vi "运维调试_总磷总氮.vi"() -> ()   [LabVIEW 2016, in "斯坦道总磷总氮.lvlib"]
uses:
  <vilib>/Utility/miscctls.llb/LVPointTypeDef.ctl
  <vilib>/Utility/config.llb/NI_LVConfig.lvlib
  <vilib>/ptbypt/NI_PtbyPt.lvlib
panel:
  in  "模块启用":bool
  in  "串口设置":bool
  in  "备用系数一键写入":bool
  in  "公式一键写入":bool
  in  "流程路径":path=path "C:/Users/Hsiao/Documents/斯坦道流程文件/流程.xml"
  in  "总磷总氮曲线模型":cluster{"X^2":dbl, "X":dbl, "B":dbl}(xcontrol)
  out "字符串 2":string
  in  "质控参数设置":bool
  in  "总氮自动测试量程配置":T1
  in  "总磷自动测试量程配置":T1
  out "温度2":sgl
  out "温度1":sgl
  out "ADC":sgl
  out "总氮稀释倍数":dbl
  out "固件版本号":string
  in  "数组":string[](array[string])
  in  "备用系数写入":bool
  in  "备用系数读取":bool
  in  "备用系数":T2
  in  "量程切换阈值写入":bool
  in  "量程切换阈值读取":bool
  in  "量程切换阈值":cluster{"阈值":dbl, "标液浓度":dbl}
  in  "参数下拉列表":enum16{"总磷", "总氮"}(ring)
  in  "量程下拉列表":enum16{"低量程", "高量程"}(ring)
  in  "测量模式下拉列表":enum16{"水样测量", "空白核查", "跨度核查", "标样核查", "加标回收"}(ring)
  in  "公式":cluster{"X^2":dbl, "X":dbl, "b":dbl}
  in  "写公式":bool
  in  "读公式":bool
  in  "返回":bool
  in  "设置":bool
  out "序列号":string="序列号"
  out "总氮测量数据":T3(xcontrol)
  out "总磷测量数据":T3(xcontrol)
  out "集成报警信息":string
  out "定时启动":bool
  out "总磷总氮运行状态":T4(xcontrol)
  in  "停止":bool
  in  "手动启动":bool
  in  "单步测试":bool
  in  "总磷氨氮调试":u16[](xcontrol)
  out "F3":sgl format="%#.6f"
  out "F2":sgl format="%#.6f"
  out "F1":sgl format="%#.6f"
  out "F0":sgl format="%#.6f"
  out "多列列表框":i32(listbox)
  # "参数设置"
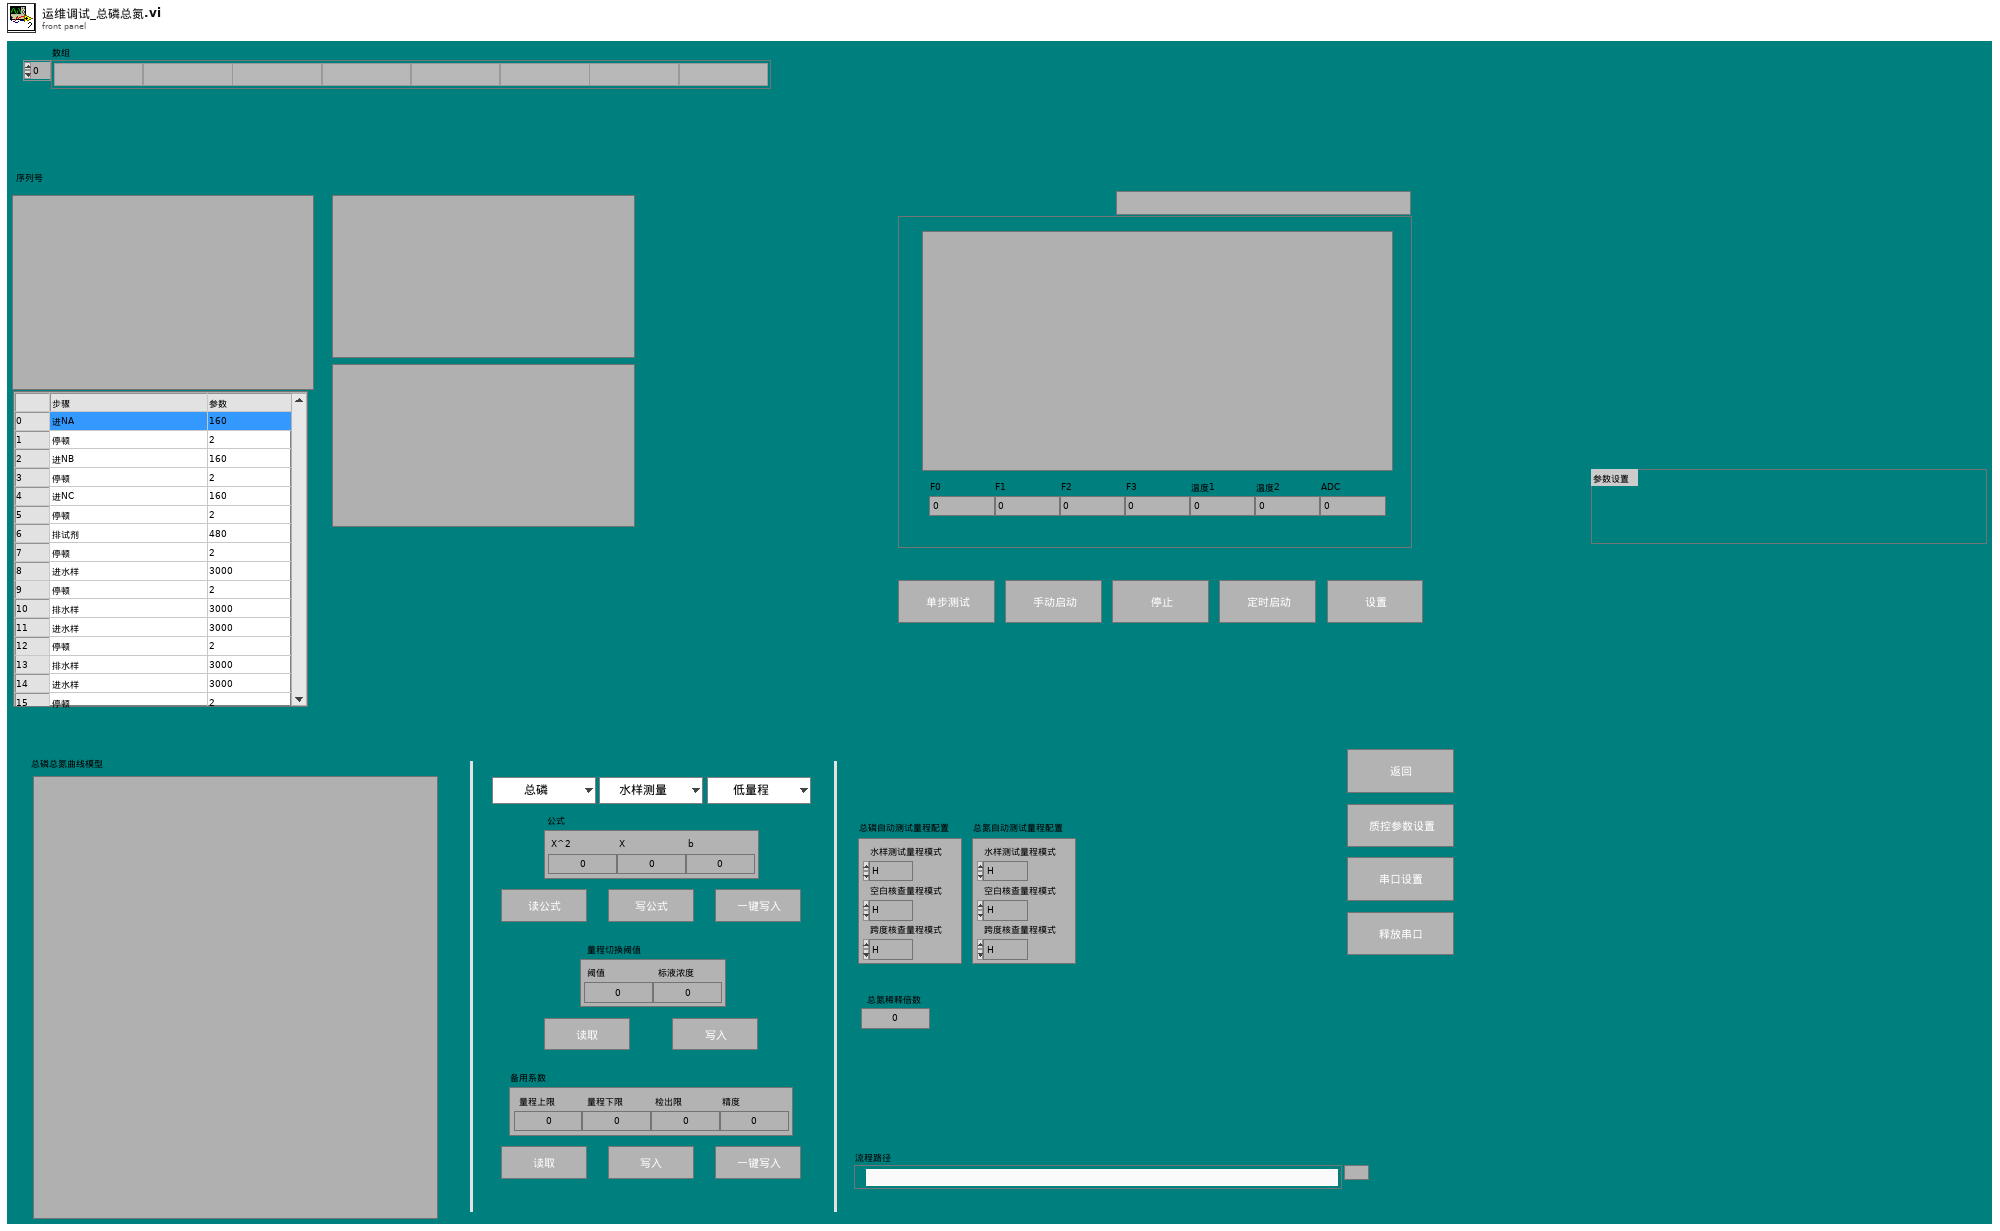
[diagram p1: front panel]
types:
  T1 = cluster{"水样测试量程模式":enum16{"H", "L", "AUTO"}, "空白核查量程模式":enum16{"H", "L", "AUTO"}, "跨度核查量程模式":enum16{"H", "L", "AUTO"}}
  T2 = cluster{"量程上限":dbl, "量程下限":dbl, "检出限":dbl, "精度":dbl}
  T3 = cluster{"flowid":u16, "测量精度":u16, "测量数据区":cluster{"因子编码":u32, "单位":u16, "标样参考值":sgl, "水样数据时间":timestamp, "水样实测值":sgl, "水样数据标识":string, "标样数据时间":timestamp, "标样实测值":sgl, "标样数据标识":string, "空白数据时间":timestamp, "空白实测值":sgl, "空白数据标识":string, "零点核查数据时间":timestamp, "零点核查实测值":sgl, "零点核查数据标识":string, "跨度核查数据时间":timestamp, "跨度核查实测值":sgl, "跨度核查数据标识":string, "加标回收数据时间":timestamp, "加标回收实测值":sgl, "加标回收数据标识":string, "平行样数据时间":timestamp, "平行样实测值":sgl, "平行样数据标识":string, "F0":sgl, "F1":sgl, "F2":sgl, "F3":sgl, "F4":sgl, "F5":sgl, "F6":sgl, "F7":sgl, "温度":sgl, "湿度":sgl, "X值":sgl}}
  T4 = cluster{"系统时间":timestamp, "工作状态":enum16{"空闲", "水样测试", "标样核查", "零点核查", "跨度核查", "空白测试", "平行样测试", "加标回收", "空白校准", "标样校准", "初始化（清洗）"}, "测量模式":enum16{"待机", "连续模式", "周期模式", "定点模式", "受控模式", "手动模式"}, "告警代码":enum16{"无告警", "缺试剂告警", "缺水样告警", "缺蒸馏水告警", "缺标液告警", "仪表漏液告警", "标定异常告警", "超量程告警", "加热异常", "低试剂预警", "超上限告警", "超下限告警", "仪表内部其他异常", "滴定异常告警", "电极异常告警", "量程切换告警", "参数设置告警", "PH电极电位异常", "电导率电极异常", "浊度光度异常", "溶解氧电极异常", "溶解氧光强异常", "温度异常告警", "PH异常告警", "溶解氧异常告警", "电导率异常告警", "浊度异常告警", "叶绿素异常告警", "藻密度异常告警", "蓝绿藻异常告警", "ORP异常告警", "氨氮异常告警", "清洁刷异常告警", "SD卡异常告警", "蓝牙异常告警", "Wifi异常告警", "流程异常告警"}, "故障代码":enum16{"无故障", "电机故障", "温度故障", "通讯故障", "滴定故障"}, "日志代码":u16, "软件版本":u16, "F0":sgl, "F1":sgl, "F2":sgl, "F3":sgl, "T":sgl, "H":sgl, "id":u16, "flowid":u16, "量程":u16, "总磷控温温度1":sgl, "营养盐控温温度2":sgl, "ADC":sgl}
  T5 = cluster{"站号":u16, "量程切换":enum32{"H", "L", "AUTO"}, "控制命令":enum16{"启动测量", "标样核查", "零点核查", "跨度核查", "空白测试", "平行样测试", "加标回收", "空白校准", "标样校准", "初始化（清洗）", "停止测试", "仪器重启", "校时", "模式设置", "测量间隔设置"}, "模式设置":enum16{"待机", "连续模式", "周期模式", "定点模式", "受控模式", "手动模式"}, "测量间隔":u16}
  T6 = enum16{"启动测量", "标样核查", "零点核查", "跨度核查", "空白测试", "平行样测试", "加标回收", "空白校准", "标样校准", "初始化（清洗）", "停止测试", "仪器重启", "校时", "模式设置", "测量间隔设置"}
  T7 = cluster{"仪器测试类型":enum16{"水样测试", "标样核查", "空白测试", "跨度核查"}, "周期设置类型":enum16{"定点启动", "间隔启动"}, "定时功能启用":bool, "定时间隔":dbl, "24H周期设置":bool[]}
  T8 = enum32{"Bad", "Idle", "Run top level", "Running"}
  T9 = typedef "LVDateTimeRec.ctl" = cluster{"秒数的小数部分":dbl, "秒":i32, "分":i32, "时":i32, "日":i32, "月":i32, "年":i32, "天数（周）":i32, "天数（年）":i32, "DST":i32}
  T10 = typedef "LVPointTypeDef.ctl" = cluster{"Horizontal":i16, "Vertical":i16}
  T11 = cluster{"因子编码":u32, "单位":u16, "标样参考值":sgl, "水样数据时间":timestamp, "水样实测值":sgl, "水样数据标识":string, "标样数据时间":timestamp, "标样实测值":sgl, "标样数据标识":string, "空白数据时间":timestamp, "空白实测值":sgl, "空白数据标识":string, "零点核查数据时间":timestamp, "零点核查实测值":sgl, "零点核查数据标识":string, "跨度核查数据时间":timestamp, "跨度核查实测值":sgl, "跨度核查数据标识":string, "加标回收数据时间":timestamp, "加标回收实测值":sgl, "加标回收数据标识":string, "平行样数据时间":timestamp, "平行样实测值":sgl, "平行样数据标识":string, "F0":sgl, "F1":sgl, "F2":sgl, "F3":sgl, "F4":sgl, "F5":sgl, "F6":sgl, "F7":sgl, "温度":sgl, "湿度":sgl, "X值":sgl}
  T12 = enum16{"空闲", "水样测试", "标样核查", "零点核查", "跨度核查", "空白测试", "平行样测试", "加标回收", "空白校准", "标样校准", "初始化（清洗）"}
  T13 = typedef "NI_LVConfig.lvlib/Config Data RefNum.ctl" = refnum<k1>
  T14 = cluster{"启动模式":enum16{"跨度核查", "水样测量", "空白核查", "标样核查", "加标回收"}, "启动参数":u16, "量程":enum16{"低量程", "高量程"}}
  T15 = cluster{"时间标识":timestamp, "设备":string, "日志信息":string, "流程参数":string}
  T16 = cluster{"时间标识":timestamp, "设备":string, "日志信息":string}
  T17 = enum16{"无告警", "缺试剂告警", "缺水样告警", "缺蒸馏水告警", "缺标液告警", "仪表漏液告警", "标定异常告警", "超量程告警", "加热异常", "低试剂预警", "超上限告警", "超下限告警", "仪表内部其他异常", "滴定异常告警", "电极异常告警", "量程切换告警", "参数设置告警", "PH电极电位异常", "电导率电极异常", "浊度光度异常", "溶解氧电极异常", "溶解氧光强异常", "温度异常告警", "PH异常告警", "溶解氧异常告警", "电导率异常告警", "浊度异常告警", "叶绿素异常告警", "藻密度异常告警", "蓝绿藻异常告警", "ORP异常告警", "氨氮异常告警", "清洁刷异常告警", "SD卡异常告警", "蓝牙异常告警", "Wifi异常告警", "流程异常告警"}
  T18 = typedef "LVRowAndColumnUnsignedTypeDef.ctl" = cluster{"Row":u32, "Column":u32}
  T19 = cluster{"总磷跨度值":dbl, "总磷零点标准液浓度":dbl, "总磷跨度标准液浓度":dbl, "总磷标准液标准浓度":dbl, "总氮跨度值":dbl, "总氮零点标准液浓度":dbl, "总氮跨度标准液浓度":dbl, "总氮标准液标准浓度":dbl}
  T20 = cluster{"确定":bool, "总磷跨度值":dbl, "总磷零点标准液浓度":dbl, "总磷跨度标准液浓度":dbl, "总磷标准液标准浓度":dbl, "总氮跨度值":dbl, "总氮零点标准液浓度":dbl, "总氮跨度标准液浓度":dbl, "总氮标准液标准浓度":dbl}
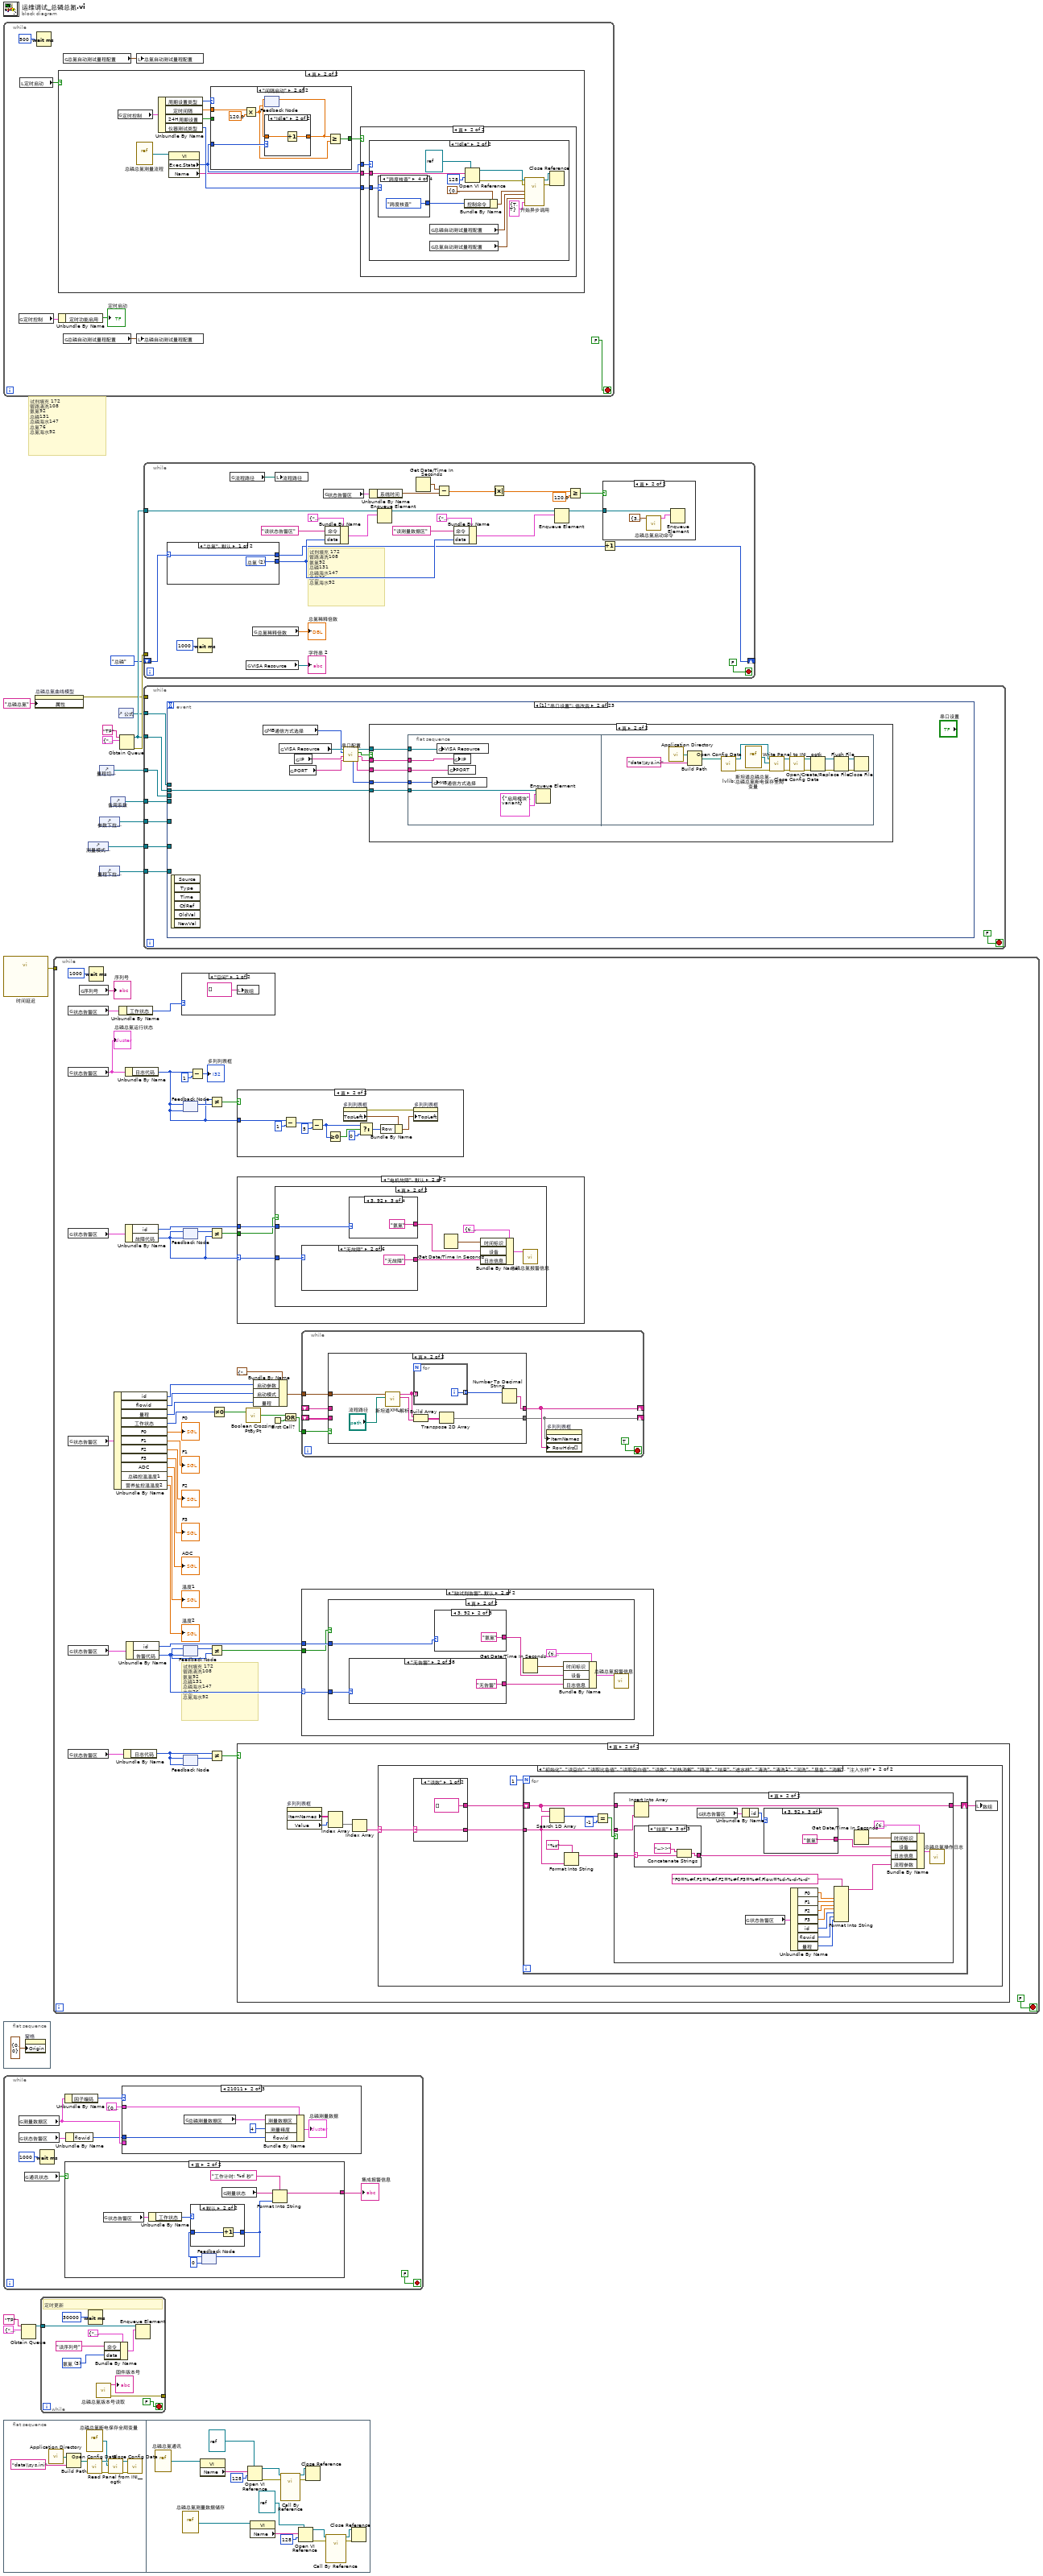
[diagram p0: block diagram]
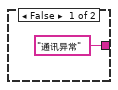
[diagram p2: hidden frame]
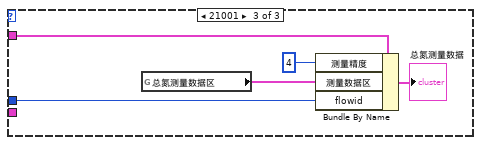
[diagram p5: hidden frame]
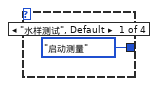
[diagram p9: hidden frame]
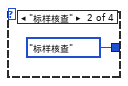
[diagram p10: hidden frame]
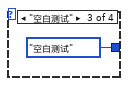
[diagram p11: hidden frame]
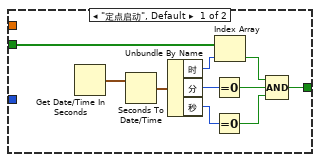
[diagram p12: hidden frame]
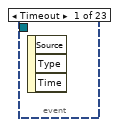
[diagram p14: hidden frame]
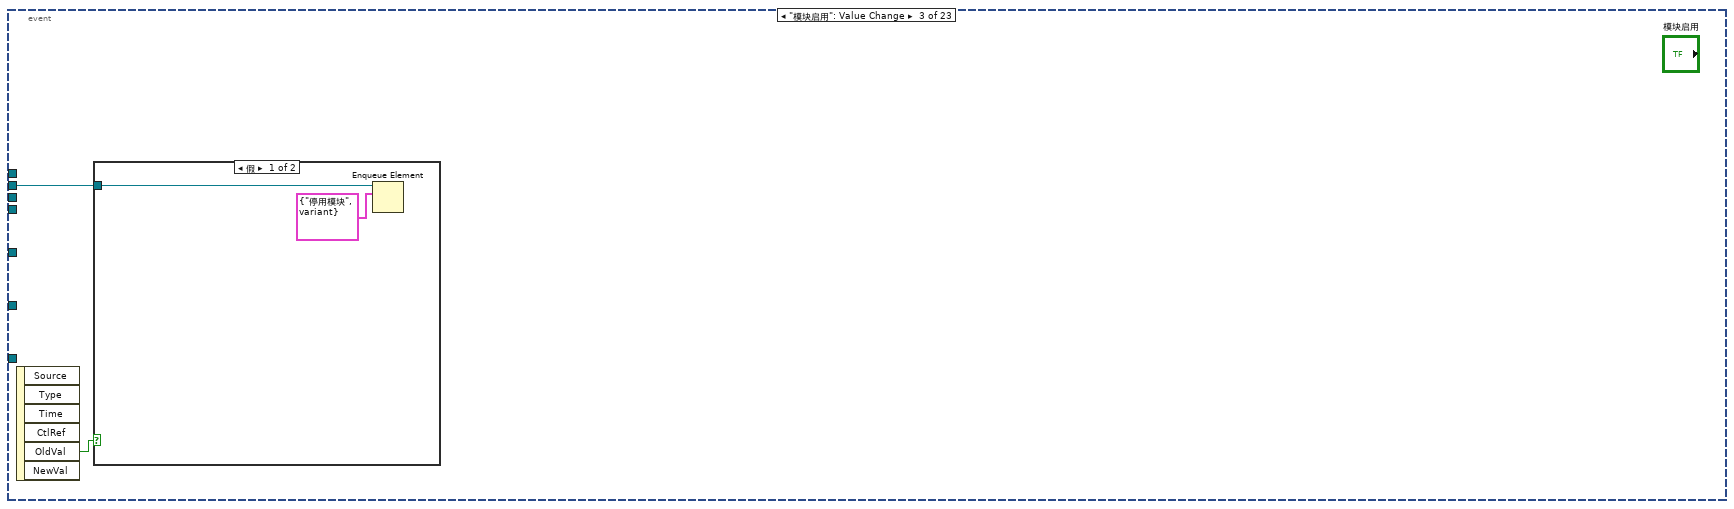
[diagram p16: hidden frame]
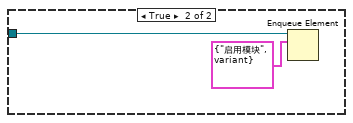
[diagram p17: hidden frame]
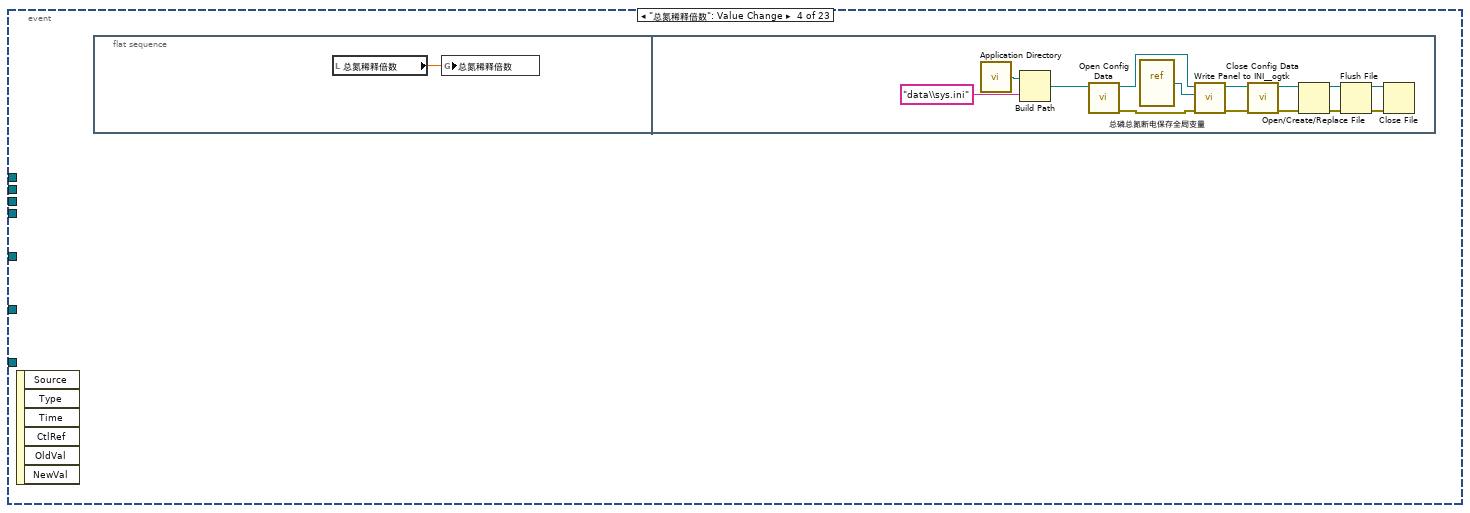
[diagram p18: hidden frame]
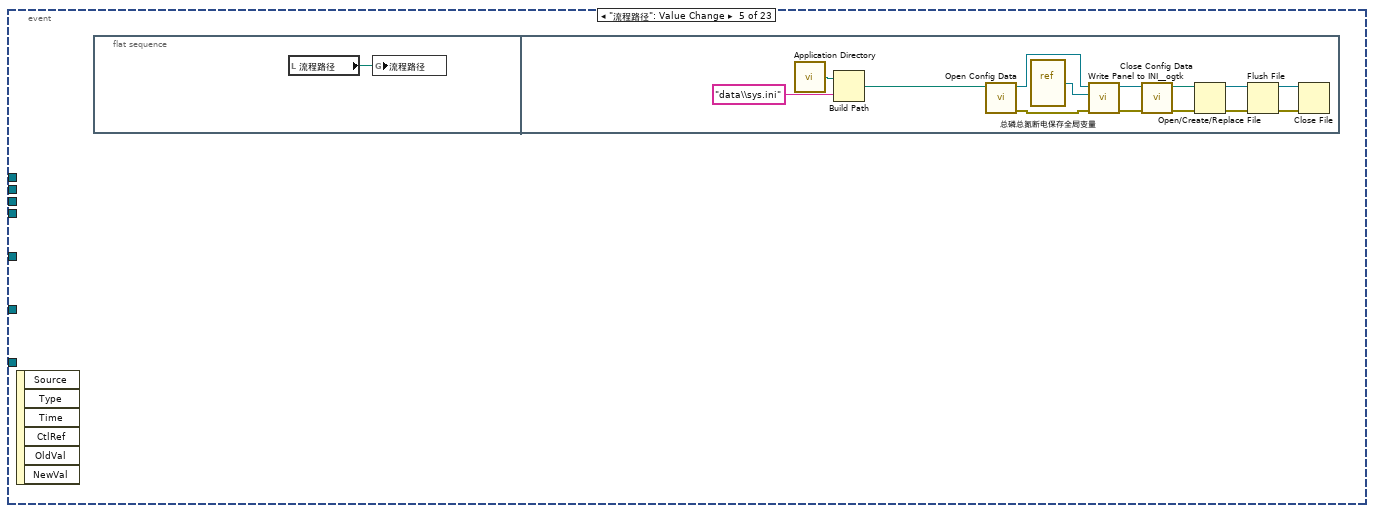
[diagram p19: hidden frame]
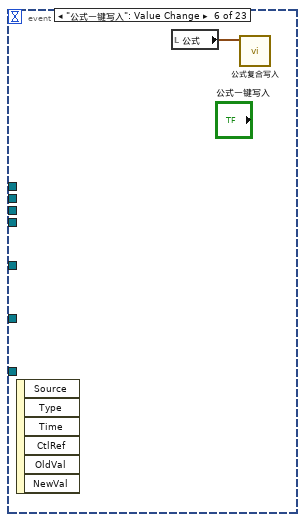
[diagram p20: hidden frame]
diagram:
  # "试剂填充 172 \n管路清洗108\n氨氮92\n总磷131\n总磷海水147\n总氮76\n总氮海水92"
  n1 = while {
    stop <- FALSE stop-if-true
    n2 = global read "总磷总氮断电保存全局变量.vi" "定时控制"() -> (w19:T7)
    n3 = local read "定时启动"() -> (w22:bool)
    n4 = Wait (ms)(milliseconds to wait=u32 500 ("等待时间（毫秒）")) -> ()  [unwired: 1 out]
    n5 = case shown="真" w22 {
      frame False {
      }
      frame True {
        n6 = global read "总磷总氮断电保存全局变量.vi" "定时控制"() -> (w33:T7)
        n7 = vi-ref "总磷总氮测量流程.vi"() -> (w28:refnum<vi>)
        n8 = Unbundle By Name(w33) -> ("周期设置类型"=w32:enum16{"定点启动", "间隔启动"}, "定时间隔"=w31:dbl, "24H周期设置"=w30:bool[], "仪器测试类型"=w27:enum16{"水样测试", "标样核查", "空白测试", "跨度核查"})
        n9 = property class="VI"(reference=w28) -> ("Exec.State"=w26:T8, "Name"=w25:string)  [unwired: 1 in, 2 out]
        n10 = case shown="\"间隔启动\"" w32 {
          tunnel: w31 -> [_ w68]
          tunnel: w30 -> [w64 _]
          tunnel: w26 -> [_ w71]
          tunnel: [w63 w66] -> w29
          frame "定点启动", Default {
            n11 = Get Date/Time In Seconds() -> (seconds since 1Jan1904=w62:timestamp)
            n12 = Seconds To Date/Time(time stamp (now)=w62) -> (date time rec=w61:T9)  [unwired: 1 in]
            n13 = Unbundle By Name(w61) -> ("时"=w60:i32, "分"=w58:i32, "秒"=w59:i32)
            n14 = Equal To 0?(x=w58) -> (x = 0?=w56:bool)
            n15 = Equal To 0?(x=w59) -> (x = 0?=w55:bool)
            n16 = Index Array(array=w64, index=w60) -> (element=w57:bool)
            n17 = Compound Arithmetic op=AND ("复合运算")(w57, w56, w55) -> (w63:bool)
          }
          frame "间隔启动" {
            n18 = Multiply(x=w68, y=120.0) -> (x*y=w65:dbl)
            n19 = feedback #1(w65) -> (w70:dbl)
            n20 = case shown="\"Idle\"" w71 {
              tunnel: w70 -> [_ w73]
              tunnel: [_ w72] -> w69
              frame "Bad", Default {
              }
              frame "Idle" {
                n21 = Increment(x=w73) -> (x+1=w72:dbl)
              }
            }
            n22 = feedback-in #1(w69) -> ()
            n23 = Greater Or Equal?(x=w69, y=w65) -> (x >= y?=w66:bool)
          }
        }
        n24 = case shown="真" w29 {
          tunnel: w25 -> [_ w36]
          tunnel: w27 -> [_ w35]
          tunnel: w26 -> [_ w34]
          frame False {
          }
          frame True {
            n25 = case shown="\"Idle\"" w34 {
              tunnel: w36 -> [_ w46]
              tunnel: w35 -> [_ w42]
              frame "Bad", Default {
              }
              frame "Idle" {
                n26 = case shown="\"跨度核查\"" w42 {
                  tunnel: [T6."启动测量" ("控制命令") T6."标样核查" ("控制命令") T6."空白测试" ("控制命令") T6."跨度核查" ("控制命令")] -> w41
                  frame "水样测试", Default {
                  }
                  frame "标样核查" {
                  }
                  frame "空白测试" {
                  }
                  frame "跨度核查" {
                  }
                }
                n27 = global read "总磷总氮断电保存全局变量.vi" "总磷自动测试量程配置"() -> (w40:T1)
                n28 = global read "总磷总氮断电保存全局变量.vi" "总氮自动测试量程配置"() -> (w39:T1)
                n29 = Bundle By Name(cluster=T5 {"站号"=0, "量程切换"=enum."H", "控制命令"=enum."启动测量", "模式设置"=enum."待机", "测量间隔"=0} ("参数"), "控制命令"=w41) -> (w43:T5)
                n30 = Open VI Reference(type specifier VI Refnum (for type only)=refnum<vi> refnum, vi path=w46, options=128 ("选项")) -> (vi reference=w47:refnum<vi>, error out=w48:errorcluster)  [unwired: 3 in]
                n31 = call-by-ref "开始异步调用"(reference=w47, error in=w48, "启动参数"=cluster{"总磷":bool, "总氮":bool} {"总磷"=TRUE, "总氮"=TRUE}, "总氮量程模式"=w39, "总磷量程模式"=w40, "参数"=w43) -> (reference out=w49:refnum<vi>, error out=w50:errorcluster)  [unwired: 8 in]
                n32 = Close Reference(reference=w49, error in (no error)=w50) -> ()  [unwired: 1 out]
              }
            }
          }
        }
      }
    }
    n33 = Unbundle By Name(w19) -> ("定时功能启用"=→"定时启动":bool)
    n34 = global read "总磷总氮断电保存全局变量.vi" "总氮自动测试量程配置"() -> (w21:T1)
    n35 = global read "总磷总氮断电保存全局变量.vi" "总磷自动测试量程配置"() -> (w20:T1)
    n36 = local write "总氮自动测试量程配置"(w21) -> ()
    n37 = local write "总磷自动测试量程配置"(w20) -> ()
  }
  n38 = call "时间延迟"() -> ("error out"=w6:errorcluster)  [unwired: 11 in]
  n39 = flat-sequence {
    frame #0 {
      n40 = property on="窗格" class="Pane"("Origin"=T10 {"Horizontal"=0, "Vertical"=0} ("原点")) -> ()  [unwired: 2 in, 2 out]
    }
  }
  n41 = while {
    stop <- FALSE stop-if-true
    n42 = global read "VAR总磷总氮全局变量.vi" "测量数据区"() -> (w81:T11)
    n43 = global read "VAR总磷总氮全局变量.vi" "状态告警区"() -> (w77:T4)
    n44 = global read "VAR总磷总氮全局变量.vi" "通讯状态"() -> (w79:bool)
    n45 = Wait (ms)(milliseconds to wait=u32 1000 ("等待时间（毫秒）")) -> ()  [unwired: 1 out]
    n46 = Unbundle By Name(w81) -> ("因子编码"=w80:u32)
    n47 = case shown="真" w79 {
      tunnel: ["通讯异常" ("集成报警信息") w86] -> w78
      frame False {
      }
      frame True {
        n48 = global read "VAR总磷总氮全局变量.vi" "状态告警区"() -> (w92:T4)
        n49 = Unbundle By Name(w92) -> ("工作状态"=w91:T12)
        n50 = feedback #2(0) -> (w89:i32)
        n51 = case shown="默认" w91 {
          tunnel: w89 -> [_ w94]
          tunnel: [_ w93] -> w87
          frame "空闲" {
          }
          frame Default {
            n52 = Increment(x=w94) -> (x+1=w93:i32)
          }
        }
        n53 = feedback-in #2(w87) -> ()
        n54 = global read "VAR总磷总氮全局变量.vi" "测量状态"() -> (w85:string)
        n55 = Format Into String(format string="工作计时: %d 秒" ("格式字符串"), initial string=w85, w87) -> (resulting string=w86:string)  [unwired: 1 in, 1 out]
      }
    }
    "集成报警信息" <- w78
    n56 = Unbundle By Name(w77) -> ("flowid"=w76:u16)
    n57 = case shown="21011" w80 {
      tunnel: w81 -> [_ _ _]
      tunnel: w76 -> [_ w97 w103]
      tunnel: T3 {"flowid"=0, "测量精度"=0, "测量数据区"={"因子编码"=0, "单位"=0, "标样参考值"=0.0, "水样数据时间"=timestamp(0 s since 1904-01-01), "水样实测值"=0.0, "水样数据标识"="", "标样数据时间"=timestamp(0 s since 1904-01-01), "标样实测值"=0.0, "标样数据标识"="", "空白数据时间"=timestamp(0 s since 1904-01-01), "空白实测值"=0.0, "空白数据标识"="", "零点核查数据时间"=timestamp(0 s since 1904-01-01), "零点核查实测值"=0.0, "零点核查数据标识"="", "跨度核查数据时间"=timestamp(0 s since 1904-01-01), "跨度核查实测值"=0.0, "跨度核查数据标识"="", "加标回收数据时间"=timestamp(0 s since 1904-01-01), "加标回收实测值"=0.0, "加标回收数据标识"="", "平行样数据时间"=timestamp(0 s since 1904-01-01), "平行样实测值"=0.0, "平行样数据标识"="", "F0"=0.0, "F1"=0.0, "F2"=0.0, "F3"=0.0, "F4"=0.0, "F5"=0.0, "F6"=0.0, "F7"=0.0, "温度"=0.0, "湿度"=0.0, "X值"=0.0}} ("总氮测量数据") -> [_ w96 w102]
      frame Default {
      }
      frame 21011 {
        n58 = global read "VAR总磷总氮全局变量.vi" "总磷测量数据区"() -> (w95:T11)
        n59 = Bundle By Name(cluster=w96, "测量数据区"=w95, "测量精度"=u16 4, "flowid"=w97) -> (→"总磷测量数据":T3)
      }
      frame 21001 {
        n60 = global read "VAR总磷总氮全局变量.vi" "总氮测量数据区"() -> (w100:T11)
        n61 = Bundle By Name(cluster=w102, "测量精度"=u16 4, "测量数据区"=w100, "flowid"=w103) -> (→"总氮测量数据":T3)
      }
    }
  }
  n62 = flat-sequence {
    frame #0 {
      n63 = call <vilib>:"Application Directory.vi"() -> ("Application Directory"=w112:path)
      n64 = Build Path(base path=w112, name or relative path="data\\sys.ini" ("名称或相对路径")) -> (appended path=w110:path)
      n65 = vi-ref "总磷总氮断电保存全局变量.vi"() -> (w108:refnum<vi>)
      n66 = call <vilib>:"Open Config Data.vi"("configuration file path"=w110) -> ("error out"=w106:errorcluster, "refnum"=w109:T13)  [unwired: 8 in, 1 out]
      n67 = call <userlib>:"Read Panel from INI__ogtk.vi"("error in (no error)"=w106, "VI ref"=w108, "refnum"=w109) -> ("error out"=w105:errorcluster, "refnum out"=w107:T13)  [unwired: 7 in]
      n68 = call <vilib>:"Close Config Data.vi"("error in (no error)"=w105, "refnum"=w107) -> ()  [unwired: 8 in, 2 out]
    }
    frame #1 {
      n69 = vi-ref "总磷总氮通讯.vi"() -> (w128:refnum<vi>)
      n70 = vi-ref "总磷总氮测量数据储存.vi"() -> (w120:refnum<vi>)
      n71 = property class="VI"(reference=w128) -> ("Name"=w127:string)  [unwired: 1 in, 2 out]
      n72 = Open VI Reference(type specifier VI Refnum (for type only)=refnum<vi> refnum, vi path=w127, options=128 ("选项")) -> (vi reference=w125:refnum<vi>, error out=w123:errorcluster)  [unwired: 3 in]
      n73 = property class="VI"(reference=w120) -> ("Name"=w113:string)  [unwired: 1 in, 2 out]
      n74 = call-by-ref "?"(reference=w125, error in=w123) -> (reference out=w121:refnum<vi>, error out=w122:errorcluster)  [unwired: 12 in]
      n75 = Open VI Reference(type specifier VI Refnum (for type only)=refnum<vi> refnum, vi path=w113, options=128 ("选项")) -> (vi reference=w115:refnum<vi>, error out=w117:errorcluster)  [unwired: 3 in]
      n76 = Close Reference(reference=w121, error in (no error)=w122) -> ()  [unwired: 1 out]
      n77 = call-by-ref "?"(reference=w115, error in=w117) -> (reference out=w119:refnum<vi>, error out=w118:errorcluster)  [unwired: 12 in]
      n78 = Close Reference(reference=w119, error in (no error)=w118) -> ()  [unwired: 1 out]
    }
  }
  n79 = Obtain Queue(name (unnamed)="TP" ("名称（未命名）"), element data type=cluster{"命令":string, "data":variant} {"命令"="", "data"=variant}) -> (queue out=w3:refnum<queue>)  [unwired: 3 in, 2 out]
  n80 = property on="总磷总氮曲线模型" class="曲线模型 (严格)"("属性"="总磷总氮" ("调用模块名称属性")) -> (error out=w1:errorcluster)  [unwired: 2 in, 1 out]
  n81 = while {
    tunnel: w3 -> [w133]
    tunnel: [w129] -> _
    stop <- FALSE stop-if-true
    w134 = u16 3 items=["总磷"=1, "氨氮"=3] ("站号")
    # "定时更新"
    n82 = Wait (ms)(milliseconds to wait=u32 30000 ("等待时间（毫秒）")) -> ()  [unwired: 1 out]
    n83 = call "总磷总氮版本号读取.vi"() -> ("error out"=w129:errorcluster, "固件版本号"=→"固件版本号":string)  [unwired: 10 in]
    n84 = Bundle By Name(cluster=cluster{"命令":string, "data":variant} {"命令"="", "data"=variant} ("元素"), "命令"="读序列号", "data"=w134) -> (w132:cluster{"命令":string, "data":variant})
    n85 = Enqueue Element(queue=w133, element=w132) -> ()  [unwired: 2 in, 3 out]
  }
  n86 = while {
    tunnel: w6 -> [_]
    stop <- FALSE stop-if-true
    # "试剂填充 172 \n管路清洗108\n氨氮92\n总磷131\n总磷海水147\n总氮76\n总氮海水92"
    n87 = global read "VAR总磷总氮全局变量.vi" "状态告警区"() -> (w152:T4)
    n88 = global read "VAR总磷总氮全局变量.vi" "状态告警区"() -> (w165:T4)
    "总磷总氮运行状态" <- w165
    n89 = global read "VAR总磷总氮全局变量.vi" "状态告警区"() -> (w157:T4)
    n90 = global read "VAR总磷总氮全局变量.vi" "状态告警区"() -> (w173:T4)
    n91 = global read "VAR总磷总氮全局变量.vi" "状态告警区"() -> (w162:T4)
    n92 = global read "VAR总磷总氮全局变量.vi" "状态告警区"() -> (w149:T4)
    n93 = global read "VAR总磷总氮全局变量.vi" "序列号"() -> (→"序列号":string)
    n94 = Wait (ms)(milliseconds to wait=u32 1000 ("等待时间（毫秒）")) -> ()  [unwired: 1 out]
    n95 = Unbundle By Name(w173) -> ("id"=w170:u16, "flowid"=w172:u16, "量程"=w171:u16, "工作状态"=w139:T12, "F0"=→"F0":sgl, "F1"=→"F1":sgl, "F2"=→"F2":sgl, "F3"=→"F3":sgl, "ADC"=→"ADC":sgl, "总磷控温温度1"=→"温度1":sgl, "营养盐控温温度2"=→"温度2":sgl)
    n96 = Unbundle By Name(w152) -> ("工作状态"=w151:T12)
    n97 = Unbundle By Name(w149) -> ("日志代码"=w148:u16)
    n98 = Unbundle By Name(w165) -> ("日志代码"=w145:u16)
    n99 = Unbundle By Name(w157) -> ("id"=w156:u16, "故障代码"=w153:enum16{"无故障", "电机故障", "温度故障", "通讯故障", "滴定故障"})
    n100 = Unbundle By Name(w162) -> ("id"=w161:u16, "告警代码"=w158:T17)
    n101 = case shown="\"空闲\"" w151 {
      frame "空闲" {
        n102 = local write "数组"(string[] [] ("数组")) -> ()
      }
      frame "水样测试", Default {
      }
    }
    n103 = feedback-in #3(w145) -> ()
    n104 = feedback #3(w145) -> (w178:u16)
    n105 = feedback #4(w153) -> (w154:enum16{"无故障", "电机故障", "温度故障", "通讯故障", "滴定故障"})
    n106 = feedback-in #4(w153) -> ()
    n107 = feedback #5(w158) -> (w159:T17)
    n108 = feedback-in #5(w158) -> ()
    n109 = feedback #6(w148) -> (w150:u16)
    n110 = feedback-in #6(w148) -> ()
    n111 = Subtract(x=w145, y=1) -> (x-y=→"多列列表框":i32)
    n112 = Not Equal?(x=w145, y=w178) -> (x != y?=w177:bool)
    n113 = Not Equal?(x=w154, y=w153) -> (x != y?=w155:bool)
    n114 = Not Equal?(x=w159, y=w158) -> (x != y?=w160:bool)
    n115 = Not Equal?(x=w148, y=w150) -> (x != y?=w147:bool)
    n116 = Not Equal To 0?(x=w139) -> (x != 0?=w175:bool)
    n117 = case shown="真" w177 {
      tunnel: w145 -> [_ w331]
      frame False {
      }
      frame True {
        n118 = Subtract(x=w331, y=1) -> (x-y=w329:i32)
        n119 = Subtract(x=w329, y=5) -> (x-y=w333:i32)
        n120 = Greater Or Equal To 0?(x=w333) -> (x >= 0?=w332:bool)
        n121 = property on="多列列表框" class="MCListbox (严格)"() -> (error out=w337:errorcluster, "TopLeft"=w338:T18)  [unwired: 2 in, 1 out]
        n122 = Select(t=w333, s=w332, f=0) -> (s? t:f=w334:i32)
        n123 = Bundle By Name(cluster=w338, "Row"=w334) -> (w339:T18)
        n124 = property on="多列列表框" class="MCListbox (严格)"(error in=w337, "TopLeft"=w339) -> ()  [unwired: 1 in, 2 out]
      }
    }
    n125 = case shown="\"电机故障\", 默认" w153 {
      selector: w153 -> [_ w236]
      tunnel: w156 -> [_ w237]
      tunnel: w155 -> [_ w235]
      frame "无故障" {
      }
      frame "电机故障", Default {
        n126 = case shown="真" w235 {
          tunnel: w237 -> [_ w244]
          tunnel: w236 -> [_ w239]
          frame False {
          }
          frame True {
            n127 = case shown="\"无故障\"" w239 {
              selector: w239 -> [w246 _ _ _ _ _]
              tunnel: [w245 "无故障" "电机故障" "温度故障" "通讯故障" "滴定故障"] -> w238
              frame Default {
                n128 = Format Into String(format string="%d" ("格式字符串"), initial string="未知" ("工作状态"), w246) -> (resulting string=w245:string)  [unwired: 1 in, 1 out]
              }
              frame "无故障" {
              }
              frame "电机故障" {
              }
              frame "温度故障" {
              }
              frame "通讯故障" {
              }
              frame "滴定故障" {
              }
            }
            n129 = case shown="3, 92" w244 {
              tunnel: [_ "总磷" ("table输入") "氨氮" ("table输入") "总氮" ("table输入")] -> w240
              frame Default {
              }
              frame 1, 131 {
              }
              frame 3, 92 {
              }
              frame 2, 76 {
              }
            }
            n130 = Get Date/Time In Seconds() -> (seconds since 1Jan1904=w241:timestamp)
            n131 = Bundle By Name(cluster=T16 {"时间标识"=timestamp(0 s since 1904-01-01), "设备"="", "日志信息"=""} ("data in"), "时间标识"=w241, "设备"=w240, "日志信息"=w238) -> (w242:T16)
            n132 = call "总磷总氮报警信息.vi"("data in"=w242) -> ()  [unwired: 11 in]
          }
        }
      }
    }
    n133 = case shown="真" w147 {
      frame False {
      }
      frame True {
        n134 = property on="多列列表框" class="MCListbox (严格)"() -> ("ItemNames"=w184:string[][], "Value"=w185:i32)  [unwired: 2 in, 2 out]
        n135 = Index Array(array=w184, index (row)=w185) -> (element=w183:string[])  [unwired: 1 in]
        n136 = Index Array(array=w183) -> (element=w182:string)  [unwired: 1 in]
        n137 = case shown="\"初始化\", \"读空白\", \"读取比色值\", \"读取空白值\", \"读数\", \"加热消解\", \"降温\", \"结束\", \"进水样\", \"清洗\", \"清洗1\", \"润洗\", \"显色\", \"消解\", \"注入水样\"" w182 {
          selector: w182 -> [_ w188]
          frame Default {
          }
          frame "初始化", "读空白", "读取比色值", "读取空白值", "读数", "加热消解", "降温", "结束", "进水样", "清洗", "清洗1", "润洗", "显色", "消解", "注入水样" {
            n138 = case shown="\"读数\"" w188 {
              selector: w188 -> [w192 w194]
              tunnel: [w192 w194] -> w187
              tunnel: [string[] [] ("数组") "数组"] -> w186
              frame "读数" {
              }
              frame Default {
              }
            }
            n139 = for {
              N: 1 -> [_]
              tunnel: w187 -> [w196]
              shift-right: [w195] -> w189
              shift-left: w186 -> [w197]
              n140 = Search 1D Array(1D array=w197, element=w196) -> (index of element=w200:i32)  [unwired: 1 in]
              n141 = Format Into String(format string="%s" ("格式字符串"), w196) -> (resulting string=w201:string)  [unwired: 2 in, 1 out]
              n142 = Equal?(x=w200, y=-1) -> (x = y?=w198:bool)
              n143 = case shown="真" w198 {
                tunnel: w201 -> [_ w205]
                tunnel: w197 -> [w203 w209]
                tunnel: w196 -> [_ w208]
                tunnel: [w203 w207] -> w195
                frame False {
                }
                frame True {
                  n144 = Insert Into Array(array=w209, new element=w208) -> (w207:string[])  [unwired: 1 in]
                  n145 = case shown="\"结束\"" w205 {
                    selector: w205 -> [w225 w228 w231]
                    tunnel: [w225 w227 w230] -> w204
                    frame Default {
                    }
                    frame "初始化" {
                      n146 = Concatenate Strings("-->>" ("字符串"), w228) -> (w227:string)
                    }
                    frame "结束" {
                      n147 = Concatenate Strings("-->>" ("字符串"), w231) -> (w230:string)
                    }
                  }
                  n148 = global read "VAR总磷总氮全局变量.vi" "状态告警区"() -> (w224:T4)
                  n149 = Unbundle By Name(w224) -> ("id"=w223:u16)
                  n150 = global read "VAR总磷总氮全局变量.vi" "状态告警区"() -> (w219:T4)
                  n151 = case shown="3, 92" w223 {
                    tunnel: [_ "总磷" ("table输入") "氨氮" ("table输入") "总氮" ("table输入")] -> w221
                    frame Default {
                    }
                    frame 1, 131 {
                    }
                    frame 3, 92 {
                    }
                    frame 2, 76 {
                    }
                  }
                  n152 = Unbundle By Name(w219) -> ("F0"=w216:sgl, "F1"=w215:sgl, "F2"=w214:sgl, "F3"=w213:sgl, "id"=w212:u16, "flowid"=w211:u16, "量程"=w210:u16)
                  n153 = Format Into String(format string="F0=%#f,F1=%#f,F2=%#f,F3=%#f,Flow=%d-%-d-%-d" ("格式字符串"), w216, w215, w214, w213, w212, w211, w210) -> (resulting string=w217:string)  [unwired: 2 in, 1 out]
                  n154 = Get Date/Time In Seconds() -> (seconds since 1Jan1904=w220:timestamp)
                  n155 = Bundle By Name(cluster=T15 {"时间标识"=timestamp(0 s since 1904-01-01), "设备"="", "日志信息"="", "流程参数"=""} ("data in"), "时间标识"=w220, "设备"=w221, "日志信息"=w204, "流程参数"=w217) -> (w222:T15)
                  n156 = call "总磷总氮操作日志.vi"("data in"=w222) -> ()  [unwired: 11 in]
                }
              }
            }
            n157 = local write "数组"(w189) -> ()
          }
        }
      }
    }
    n158 = call <vilib>:"Boolean Crossing PtByPt.vi"("input"=w175) -> ("crossing"=w138:bool)  [unwired: 2 in]
    n159 = Bundle By Name(cluster=T14 {"启动模式"=enum."跨度核查", "启动参数"=1, "量程"=enum."低量程"} ("参数簇"), "启动参数"=w170, "启动模式"=w172, "量程"=w171) -> (w164:T14)
    n160 = First Call?() -> (First Call?: T/F=w176:bool)
    n161 = Or(x=w138, y=w176) -> (x .or. y?=w174:bool)
    n162 = while {
      tunnel: w174 -> [w317]
      tunnel: w164 -> [w316]
      shift-right: [w311] -> _
      shift-left: _ -> [w313]
      shift-right: [w312] -> _
      shift-left: _ -> [w314]
      stop <- TRUE stop-if-true
      n163 = case shown="真" w317 {
        tunnel: [w319 w327] -> w312
        tunnel: [w318 w326] -> w311
        tunnel: w316 -> [_ w321]
        tunnel: w314 -> [w319 _]
        tunnel: w313 -> [w318 _]
        frame False {
        }
        frame True {
          n164 = call "斯坦道XML解析.vi"("添加的路径"="流程路径", "参数簇"=w321) -> ("步骤时间"=w322:string[], "步骤名"=w324:string[])  [unwired: 8 in]
          n165 = for {
            tunnel: w324 -> [_] mode=indexing
            tunnel: [w328] -> w325 mode=indexing
            i -> [w328]
          }
          n166 = Build Array(w324, w322) -> (w323:string[][])
          n167 = Transpose 2D Array(2D array=w323) -> (transposed array=w326:string[][])
          n168 = Number To Decimal String(number=w325) -> (decimal integer string=w327:string[])  [unwired: 1 in]
        }
      }
      n169 = property on="多列列表框" class="MCListbox (严格)"("ItemNames"=w311, "RowHdrs[]"=w312) -> ()  [unwired: 2 in, 2 out]
    }
    n170 = case shown="\"缺试剂告警\", 默认" w158 {
      selector: w158 -> [_ w258]
      tunnel: w161 -> [_ w259]
      tunnel: w160 -> [_ w257]
      frame "无告警" {
      }
      frame "缺试剂告警", Default {
        n171 = case shown="真" w257 {
          tunnel: w259 -> [_ w266]
          tunnel: w258 -> [_ w260]
          frame False {
          }
          frame True {
            n172 = case shown="\"无告警\"" w260 {
              selector: w260 -> [w268 _ _ _ _ _ _ _ _ _ _ _ _ _ _ _ _ _ _ _ _ _ _ _ _ _ _ _ _ _ _ _ _ _ _ _ _ _]
              tunnel: [w267 "无告警" "缺试剂告警" "缺水样告警" "缺蒸馏水告警" "缺标液告警" "仪表漏液告警" "标定异常告警" "超量程告警" "加热异常" "低试剂预警" "超上限告警" "超下限告警" "仪表内部其他异常" "滴定异常告警" "电极异常告警" "量程切换告警" "参数设置告警" "PH电极电位异常" "电导率电极异常" "浊度光度异常" "溶解氧电极异常" "溶解氧光强异常" "温度异常告警" "PH异常告警" "溶解氧异常告警" "电导率异常告警" "浊度异常告警" "叶绿素异常告警" "藻密度异常告警" "蓝绿藻异常告警" "ORP异常告警" "氨氮异常告警" "清洁刷异常告警" "SD卡异常告警" "蓝牙异常告警" "WiFi异常告警" "流程异常告警"] -> w261
              frame Default {
                n173 = Format Into String(format string="%d" ("格式字符串"), initial string="未知" ("工作状态"), w268) -> (resulting string=w267:string)  [unwired: 1 in, 1 out]
              }
              frame "无告警" {
              }
              frame "缺试剂告警" {
              }
              frame "缺水样告警" {
              }
              frame "缺蒸馏水告警" {
              }
              frame "缺标液告警" {
              }
              frame "仪表漏液告警" {
              }
              frame "标定异常告警" {
              }
              frame "超量程告警" {
              }
              frame "加热异常" {
              }
              frame "低试剂预警" {
              }
              frame "超上限告警" {
              }
              frame "超下限告警" {
              }
              frame "仪表内部其他异常" {
              }
              frame "滴定异常告警" {
              }
              frame "电极异常告警" {
              }
              frame "量程切换告警" {
              }
              frame "参数设置告警" {
              }
              frame "PH电极电位异常" {
              }
              frame "电导率电极异常" {
              }
              frame "浊度光度异常" {
              }
              frame "溶解氧电极异常" {
              }
              frame "溶解氧光强异常" {
              }
              frame "温度异常告警" {
              }
              frame "PH异常告警" {
              }
              frame "溶解氧异常告警" {
              }
              frame "电导率异常告警" {
              }
              frame "浊度异常告警" {
              }
              frame "叶绿素异常告警" {
              }
              frame "藻密度异常告警" {
              }
              frame "蓝绿藻异常告警" {
              }
              frame "ORP异常告警" {
              }
              frame "氨氮异常告警" {
              }
              frame "清洁刷异常告警" {
              }
              frame "SD卡异常告警" {
              }
              frame "蓝牙异常告警" {
              }
              frame "Wifi异常告警" {
              }
              frame "流程异常告警" {
              }
            }
            n174 = case shown="3, 92" w266 {
              tunnel: ["总磷" ("table输入") "氨氮" ("table输入") "总氮" ("table输入")] -> w262
              frame 1, 131 {
              }
              frame 3, 92 {
              }
              frame 2, 76, Default {
              }
            }
            n175 = Get Date/Time In Seconds() -> (seconds since 1Jan1904=w263:timestamp)
            n176 = Bundle By Name(cluster=T16 {"时间标识"=timestamp(0 s since 1904-01-01), "设备"="", "日志信息"=""} ("data in"), "时间标识"=w263, "设备"=w262, "日志信息"=w261) -> (w264:T16)
            n177 = call "总磷总氮报警信息.vi"("data in"=w264) -> ()  [unwired: 11 in]
          }
        }
      }
    }
  }
  n178 = control-ref of="测量模式下拉列表"() -> (w10:refnum<vi>)
  n179 = control-ref of="量程切换阈值"() -> (w8:refnum<vi>)
  n180 = control-ref of="参数下拉列表"() -> (w11:refnum<vi>)
  n181 = control-ref of="量程下拉列表"() -> (w12:refnum<vi>)
  n182 = control-ref of="备用系数"() -> (w7:refnum<vi>)
  n183 = control-ref of="公式"() -> (w9:refnum<vi>)
  n184 = Obtain Queue(name (unnamed)="TP" ("名称（未命名）"), element data type=cluster{"命令":string, "data":variant} {"命令"="", "data"=variant}) -> (queue out=w14:refnum<queue>, error out=w15:errorcluster)  [unwired: 3 in, 1 out]
  n185 = while {
    tunnel: w14 -> [w359]
    tunnel: w15 -> [_]
    shift-right: [w351] -> _
    shift-left: enum16{"总磷", "总氮"}."总磷" ("枚举") -> [w353]
    stop <- FALSE stop-if-true
    # "试剂填充 172 \n管路清洗108\n氨氮92\n总磷131\n总磷海水147\n总氮76\n总氮海水92"
    n186 = case shown="\"总氮\", 默认" w353 {
      selector: w353 -> [w368 w370]
      tunnel: [w369 w371] -> w354
      tunnel: [w368 w370] -> w352
      frame "总氮", Default {
        w369 = u16 2 items=["总磷"=1, "总氮"=2] ("站号")
      }
      frame "总磷" {
        w371 = u16 1 items=["总磷"=1, "氨氮"=3] ("站号")
      }
    }
    n187 = Wait (ms)(milliseconds to wait=u32 1000 ("等待时间（毫秒）")) -> ()  [unwired: 1 out]
    n188 = global read "总磷总氮断电保存全局变量.vi" "流程路径"() -> (w342:path)
    n189 = global read "总磷总氮断电保存全局变量.vi" "VISA Resource"() -> (→"字符串 2":refnum<visa-resource-name>)
    n190 = global read "总磷总氮断电保存全局变量.vi" "总氮稀释倍数"() -> (→"总氮稀释倍数":dbl)
    n191 = local write "流程路径"(w342) -> ()
    n192 = global read "VAR总磷总氮全局变量.vi" "状态告警区"() -> (w343:T4)
    n193 = Bundle By Name(cluster=cluster{"命令":string, "data":variant} {"命令"="", "data"=variant} ("元素"), "命令"="读状态告警区", "data"=w354) -> (w361:cluster{"命令":string, "data":variant})
    n194 = Unbundle By Name(w343) -> ("系统时间"=w350:timestamp)
    n195 = Enqueue Element(queue=w359, element=w361) -> (queue out=w355:refnum<queue>)  [unwired: 2 in, 2 out]
    n196 = Get Date/Time In Seconds() -> (seconds since 1Jan1904=w349:timestamp)
    n197 = Subtract(x=w349, y=w350) -> (x-y=w348:dbl)
    n198 = Bundle By Name(cluster=cluster{"命令":string, "data":variant} {"命令"="", "data"=variant} ("元素"), "命令"="读测量数据区", "data"=w354) -> (w357:cluster{"命令":string, "data":variant})
    n199 = Absolute Value(x=w348) -> (abs(x)=w347:dbl)
    n200 = Enqueue Element(queue=w355, element=w357) -> (queue out=w344:refnum<queue>)  [unwired: 2 in, 2 out]
    n201 = Greater Or Equal?(x=w347, y=120.0) -> (x >= y?=w345:bool)
    n202 = case shown="真" w345 {
      tunnel: w344 -> [_ w366]
      frame False {
      }
      frame True {
        n203 = call "总磷总氮启动命令.vi"("参数"=T5 {"站号"=3, "量程切换"=enum."AUTO", "控制命令"=enum."校时", "模式设置"=enum."待机", "测量间隔"=0}) -> ("启动命令"=w365:cluster{"命令":string, "data":variant})  [unwired: 10 in]
        n204 = Enqueue Element(queue=w366, element=w365) -> ()  [unwired: 2 in, 3 out]
      }
    }
    n205 = Increment(x=w352) -> (x+1=w351:enum16{"总磷", "总氮"})
  }
  n206 = while {
    tunnel: w14 -> [w378]
    tunnel: w12 -> [w377]
    tunnel: w11 -> [w376]
    tunnel: w10 -> [w375]
    tunnel: w9 -> [w374]
    tunnel: w8 -> [w373]
    tunnel: w7 -> [w372]
    tunnel: w1 -> [_]
    stop <- FALSE stop-if-true
    n207 = event shown="[1] \"串口设置\": 值改变" {
      selector: _ -> [_ _ _ _ _ _ _ _ _ _ _ _ _ _ _ _ _ _ _ _ _ _ _]
      dyn-events: _ -> [_ _ _ _ _ _ _ _ _ _ _ _ _ _ _ _ _ _ _ _ _ _ _]
      timeout: _ -> [_ _ _ _ _ _ _ _ _ _ _ _ _ _ _ _ _ _ _ _ _ _ _]
      tunnel: w378 -> [_ w389 w415 _ _ _ _ _ _ _ w502 _ w527 w531 _ _ _ _ _ _ _ _ _]
      tunnel: w377 -> [_ _ _ _ _ _ _ _ _ _ _ _ _ _ _ _ _ w547 _ w567 w576 _ _]
      tunnel: w376 -> [_ _ _ _ _ _ _ _ _ _ _ _ _ _ _ _ _ w545 _ w565 w578 w586 w593]
      tunnel: w375 -> [_ _ _ _ _ _ _ _ _ _ _ _ _ _ _ _ _ w546 _ w566 w577 _ _]
      tunnel: w374 -> [_ _ _ _ _ _ _ _ _ _ _ _ _ _ _ _ _ w541 _ _ _ _ _]
      tunnel: w373 -> [_ _ _ _ _ _ _ _ _ _ _ _ _ _ _ _ _ _ _ w561 _ _ _]
      tunnel: w372 -> [_ _ _ _ _ _ _ _ _ _ _ _ _ _ _ _ _ _ _ _ _ w584 _]
      event Timeout {
        n208 = event-data() -> ()  [unwired: 1 in, 3 out]
      }
      event "串口设置": Value Change {
        n209 = event-data() -> ()  [unwired: 1 in, 6 out]
        n210 = global read "总磷总氮断电保存全局变量.vi" "MB通信方式选择"() -> (w380:enum16{"串口", "TCP"})
        n211 = global read "总磷总氮断电保存全局变量.vi" "VISA Resource"() -> (w386:refnum<visa-resource-name>)
        n212 = global read "总磷总氮断电保存全局变量.vi" "PORT"() -> (w384:string)
        n213 = global read "总磷总氮断电保存全局变量.vi" "IP"() -> (w385:string)
        n214 = call "串口配置.vi"("PORT"=w384, "IP"=w385, "MB通信方式选择"=w380, "请选择串口:"=w386) -> ("PORT 2"=w382:string, "IP 2"=w383:string, "确认 2"=w387:bool, "VISA资源名称 2"=w388:refnum<visa-resource-name>, "MB通信方式选择 2"=w381:enum16{"串口", "TCP"})  [unwired: 3 in]
        n215 = case shown="真" w387 {
          tunnel: w388 -> [_ w394]
          tunnel: w389 -> [_ w393]
          tunnel: w383 -> [_ w392]
          tunnel: w382 -> [_ w391]
          tunnel: w381 -> [_ w390]
          frame False {
          }
          frame True {
            n216 = flat-sequence {
              tunnel: w394 -> [w398]
              tunnel: w393 -> [w399]
              tunnel: w392 -> [w397]
              tunnel: w391 -> [w396]
              tunnel: w390 -> [w395]
              frame #0 {
                n217 = global write "总磷总氮断电保存全局变量.vi" "MB通信方式选择"(w395) -> ()
                n218 = global write "总磷总氮断电保存全局变量.vi" "VISA Resource"(w398) -> ()
                n219 = global write "总磷总氮断电保存全局变量.vi" "PORT"(w396) -> ()
                n220 = global write "总磷总氮断电保存全局变量.vi" "IP"(w397) -> ()
                n221 = Enqueue Element(queue=w399, element=cluster{"命令":string, "data":variant} {"命令"="启用模块", "data"=variant} ("元素")) -> ()  [unwired: 2 in, 3 out]
              }
              frame #1 {
                n222 = call <vilib>:"Application Directory.vi"() -> ("Application Directory"=w414:path)
                n223 = Build Path(base path=w414, name or relative path="data\\sys.ini" ("名称或相对路径")) -> (appended path=w412:path)
                n224 = call <vilib>:"Open Config Data.vi"("configuration file path"=w412) -> ("error out"=w408:errorcluster, "refnum"=w411:T13)  [unwired: 8 in, 1 out]
                n225 = vi-ref "斯坦道总磷总氮.lvlib:总磷总氮断电保存全局变量.vi"() -> (w410:refnum<vi>)
                n226 = call <userlib>:"Write Panel to INI__ogtk.vi"("error in (no error)"=w408, "VI ref"=w410, "refnum"=w411) -> ("error out"=w407:errorcluster, "refnum out"=w409:T13)  [unwired: 7 in]
                n227 = call <vilib>:"Close Config Data.vi"("error in (no error)"=w407, "refnum"=w409) -> ("error out"=w402:errorcluster, "file path"=w401:path)  [unwired: 8 in]
                n228 = Open/Create/Replace File(file path (use dialog)=w401, error in=w402) -> (refnum out=w405:refnum<file>, error out=w406:errorcluster)  [unwired: 4 in, 1 out]
                n229 = Flush File(refnum=w405, error in=w406) -> (refnum out=w404:refnum<file>, error out=w403:errorcluster)
                n230 = Close File(refnum=w404, error in=w403) -> ()  [unwired: 2 out]
              }
            }
          }
        }
      }
      event "模块启用": Value Change {
        n231 = event-data() -> ("OldVal"=w416:bool)  [unwired: 1 in, 5 out]
        n232 = case shown="假" w416 {
          tunnel: w415 -> [w417 w419]
          frame False {
            n233 = Enqueue Element(queue=w417, element=cluster{"命令":string, "data":variant} {"命令"="停用模块", "data"=variant} ("元素")) -> ()  [unwired: 2 in, 3 out]
          }
          frame True {
            n234 = Enqueue Element(queue=w419, element=cluster{"命令":string, "data":variant} {"命令"="启用模块", "data"=variant} ("元素")) -> ()  [unwired: 2 in, 3 out]
          }
        }
      }
      event "总氮稀释倍数": Value Change {
        n235 = event-data() -> ()  [unwired: 1 in, 6 out]
        n236 = flat-sequence {
          frame #0 {
            n237 = local read "总氮稀释倍数"() -> (w421:dbl)
            n238 = global write "总磷总氮断电保存全局变量.vi" "总氮稀释倍数"(w421) -> ()
          }
          frame #1 {
            n239 = call <vilib>:"Application Directory.vi"() -> ("Application Directory"=w435:path)
            n240 = Build Path(base path=w435, name or relative path="data\\sys.ini" ("名称或相对路径")) -> (appended path=w433:path)
            n241 = call <vilib>:"Open Config Data.vi"("configuration file path"=w433) -> ("error out"=w429:errorcluster, "refnum"=w432:T13)  [unwired: 8 in, 1 out]
            n242 = vi-ref "总磷总氮断电保存全局变量.vi"() -> (w431:refnum<vi>)
            n243 = call <userlib>:"Write Panel to INI__ogtk.vi"("error in (no error)"=w429, "VI ref"=w431, "refnum"=w432) -> ("error out"=w428:errorcluster, "refnum out"=w430:T13)  [unwired: 7 in]
            n244 = call <vilib>:"Close Config Data.vi"("error in (no error)"=w428, "refnum"=w430) -> ("error out"=w423:errorcluster, "file path"=w422:path)  [unwired: 8 in]
            n245 = Open/Create/Replace File(file path (use dialog)=w422, error in=w423) -> (refnum out=w426:refnum<file>, error out=w427:errorcluster)  [unwired: 4 in, 1 out]
            n246 = Flush File(refnum=w426, error in=w427) -> (refnum out=w425:refnum<file>, error out=w424:errorcluster)
            n247 = Close File(refnum=w425, error in=w424) -> ()  [unwired: 2 out]
          }
        }
      }
      event "流程路径": Value Change {
        n248 = event-data() -> ()  [unwired: 1 in, 6 out]
        n249 = flat-sequence {
          frame #0 {
            n250 = local read "流程路径"() -> (w436:path)
            n251 = global write "总磷总氮断电保存全局变量.vi" "流程路径"(w436) -> ()
          }
          frame #1 {
            n252 = call <vilib>:"Application Directory.vi"() -> ("Application Directory"=w450:path)
            n253 = Build Path(base path=w450, name or relative path="data\\sys.ini" ("名称或相对路径")) -> (appended path=w448:path)
            n254 = call <vilib>:"Open Config Data.vi"("configuration file path"=w448) -> ("error out"=w444:errorcluster, "refnum"=w447:T13)  [unwired: 8 in, 1 out]
            n255 = vi-ref "总磷总氮断电保存全局变量.vi"() -> (w446:refnum<vi>)
            n256 = call <userlib>:"Write Panel to INI__ogtk.vi"("error in (no error)"=w444, "VI ref"=w446, "refnum"=w447) -> ("error out"=w443:errorcluster, "refnum out"=w445:T13)  [unwired: 7 in]
            n257 = call <vilib>:"Close Config Data.vi"("error in (no error)"=w443, "refnum"=w445) -> ("error out"=w438:errorcluster, "file path"=w437:path)  [unwired: 8 in]
            n258 = Open/Create/Replace File(file path (use dialog)=w437, error in=w438) -> (refnum out=w441:refnum<file>, error out=w442:errorcluster)  [unwired: 4 in, 1 out]
            n259 = Flush File(refnum=w441, error in=w442) -> (refnum out=w440:refnum<file>, error out=w439:errorcluster)
            n260 = Close File(refnum=w440, error in=w439) -> ()  [unwired: 2 out]
          }
        }
      }
      event "公式一键写入": Value Change {
        n261 = event-data() -> ()  [unwired: 1 in, 6 out]
        n262 = local read "公式"() -> (w451:cluster{"X^2":dbl, "X":dbl, "b":dbl})
        n263 = call "公式复合写入.vi"("公式"=w451) -> ()  [unwired: 11 in]
      }
      event "备用系数一键写入": Value Change {
        n264 = event-data() -> ()  [unwired: 1 in, 6 out]
        n265 = local read "备用系数"() -> (w452:T2)
        n266 = call "量程参数复合参数写入.vi"("备用系数"=w452) -> ()  [unwired: 11 in]
      }
      event "总磷总氮曲线模型": Value Change {
        n267 = event-data() -> ()  [unwired: 1 in, 6 out]
        n268 = local write "公式"("总磷总氮曲线模型") -> ()
      }
      event "质控参数设置": Value Change {
        n269 = event-data() -> ()  [unwired: 1 in, 6 out]
        n270 = global read "总磷总氮断电保存全局变量.vi" "质控参数设置"() -> (w454:T19)
        n271 = call "总磷总氮质控参数设置.vi"("质控参数设置"=w454) -> ("输出簇"=w455:T20)  [unwired: 10 in]
        n272 = Unbundle By Name(w455) -> ("确定"=w456:bool)
        n273 = case shown="真" w456 {
          tunnel: w455 -> [_ w458]
          tunnel: w454 -> [_ w457]
          frame False {
          }
          frame True {
            n274 = flat-sequence {
              tunnel: w458 -> [w469]
              tunnel: w457 -> [w468]
              frame #0 {
                n275 = Unbundle By Name(w469) -> ("总磷跨度值"=w467:dbl, "总磷零点标准液浓度"=w466:dbl, "总磷跨度标准液浓度"=w465:dbl, "总磷标准液标准浓度"=w464:dbl, "总氮跨度值"=w463:dbl, "总氮零点标准液浓度"=w462:dbl, "总氮跨度标准液浓度"=w461:dbl, "总氮标准液标准浓度"=w460:dbl)
                n276 = Bundle By Name(cluster=w468, "总磷跨度值"=w467, "总磷零点标准液浓度"=w466, "总磷跨度标准液浓度"=w465, "总磷标准液标准浓度"=w464, "总氮跨度值"=w463, "总氮零点标准液浓度"=w462, "总氮跨度标准液浓度"=w461, "总氮标准液标准浓度"=w460) -> (w459:T19)
                n277 = global write "总磷总氮断电保存全局变量.vi" "质控参数设置"(w459) -> ()
              }
              frame #1 {
                n278 = call <vilib>:"Application Directory.vi"() -> ("Application Directory"=w483:path)
                n279 = Build Path(base path=w483, name or relative path="data\\sys.ini" ("名称或相对路径")) -> (appended path=w481:path)
                n280 = call <vilib>:"Open Config Data.vi"("configuration file path"=w481) -> ("error out"=w477:errorcluster, "refnum"=w480:T13)  [unwired: 8 in, 1 out]
                n281 = vi-ref "总磷总氮断电保存全局变量.vi"() -> (w479:refnum<vi>)
                n282 = call <userlib>:"Write Panel to INI__ogtk.vi"("error in (no error)"=w477, "VI ref"=w479, "refnum"=w480) -> ("error out"=w476:errorcluster, "refnum out"=w478:T13)  [unwired: 7 in]
                n283 = call <vilib>:"Close Config Data.vi"("error in (no error)"=w476, "refnum"=w478) -> ("error out"=w471:errorcluster, "file path"=w470:path)  [unwired: 8 in]
                n284 = Open/Create/Replace File(file path (use dialog)=w470, error in=w471) -> (refnum out=w474:refnum<file>, error out=w475:errorcluster)  [unwired: 4 in, 1 out]
                n285 = Flush File(refnum=w474, error in=w475) -> (refnum out=w473:refnum<file>, error out=w472:errorcluster)
                n286 = Close File(refnum=w473, error in=w472) -> ()  [unwired: 2 out]
              }
            }
          }
        }
      }
      event "总磷自动测试量程配置", "总氮自动测试量程配置": Value Change {
        n287 = event-data() -> ()  [unwired: 1 in, 6 out]
        n288 = flat-sequence {
          frame #0 {
            n289 = global write "总磷总氮断电保存全局变量.vi" "总氮自动测试量程配置"("总氮自动测试量程配置") -> ()
            n290 = global write "总磷总氮断电保存全局变量.vi" "总磷自动测试量程配置"("总磷自动测试量程配置") -> ()
          }
          frame #1 {
            n291 = call <vilib>:"Application Directory.vi"() -> ("Application Directory"=w499:path)
            n292 = Build Path(base path=w499, name or relative path="data\\sys.ini" ("名称或相对路径")) -> (appended path=w497:path)
            n293 = call <vilib>:"Open Config Data.vi"("configuration file path"=w497) -> ("error out"=w493:errorcluster, "refnum"=w496:T13)  [unwired: 8 in, 1 out]
            n294 = vi-ref "总磷总氮断电保存全局变量.vi"() -> (w495:refnum<vi>)
            n295 = call <userlib>:"Write Panel to INI__ogtk.vi"("error in (no error)"=w493, "VI ref"=w495, "refnum"=w496) -> ("error out"=w492:errorcluster, "refnum out"=w494:T13)  [unwired: 7 in]
            n296 = call <vilib>:"Close Config Data.vi"("error in (no error)"=w492, "refnum"=w494) -> ("error out"=w487:errorcluster, "file path"=w486:path)  [unwired: 8 in]
            n297 = Open/Create/Replace File(file path (use dialog)=w486, error in=w487) -> (refnum out=w490:refnum<file>, error out=w491:errorcluster)  [unwired: 4 in, 1 out]
            n298 = Flush File(refnum=w490, error in=w491) -> (refnum out=w489:refnum<file>, error out=w488:errorcluster)
            n299 = Close File(refnum=w489, error in=w488) -> ()  [unwired: 2 out]
          }
        }
      }
      event "手动启动": Value Change {
        n300 = event-data() -> ()  [unwired: 1 in, 6 out]
        n301 = call "总磷总氮启动参数对话框.vi"() -> ("确认"=w500:bool, "元素"=w501:cluster{"命令":string, "data":variant})  [unwired: 10 in]
        n302 = case shown="真" w500 {
          tunnel: w502 -> [_ w504]
          tunnel: w501 -> [_ w503]
          frame False {
          }
          frame True {
            n303 = Enqueue Element(queue=w504, element=w503) -> ()  [unwired: 2 in, 3 out]
          }
        }
      }
      event "定时启动": Mouse Down {
        n304 = event-data() -> ()  [unwired: 1 in, 6 out]
        n305 = flat-sequence {
          frame #0 {
            n306 = global read "总磷总氮断电保存全局变量.vi" "定时控制"() -> (w506:T7)
            n307 = call "总磷总氮周期设置.vi"("定时控制参数输入"=w506) -> ("定时控制参数输出"=w505:T7)  [unwired: 10 in]
            n308 = global write "总磷总氮断电保存全局变量.vi" "定时控制"(w505) -> ()
          }
          frame #1 {
            n309 = call <vilib>:"Application Directory.vi"() -> ("Application Directory"=w520:path)
            n310 = Build Path(base path=w520, name or relative path="data\\sys.ini" ("名称或相对路径")) -> (appended path=w518:path)
            n311 = call <vilib>:"Open Config Data.vi"("configuration file path"=w518) -> ("error out"=w514:errorcluster, "refnum"=w517:T13)  [unwired: 8 in, 1 out]
            n312 = vi-ref "总磷总氮断电保存全局变量.vi"() -> (w516:refnum<vi>)
            n313 = call <userlib>:"Write Panel to INI__ogtk.vi"("error in (no error)"=w514, "VI ref"=w516, "refnum"=w517) -> ("error out"=w513:errorcluster, "refnum out"=w515:T13)  [unwired: 7 in]
            n314 = call <vilib>:"Close Config Data.vi"("error in (no error)"=w513, "refnum"=w515) -> ("error out"=w508:errorcluster, "file path"=w507:path)  [unwired: 8 in]
            n315 = Open/Create/Replace File(file path (use dialog)=w507, error in=w508) -> (refnum out=w511:refnum<file>, error out=w512:errorcluster)  [unwired: 4 in, 1 out]
            n316 = Flush File(refnum=w511, error in=w512) -> (refnum out=w510:refnum<file>, error out=w509:errorcluster)
            n317 = Close File(refnum=w510, error in=w509) -> ()  [unwired: 2 out]
          }
        }
      }
      event "单步测试": Value Change {
        w522 = u16 1 items=["总磷"=1, "氨氮"=3] ("站号")
        n318 = event-data() -> ()  [unwired: 1 in, 6 out]
        n319 = Bundle("站号"=w522, "总磷氨氮调试"="总磷氨氮调试") -> (w521:cluster{"站号":u16, "总磷氨氮调试":u16[]})  [unwired: 1 in]
        n320 = Bundle By Name(cluster=cluster{"命令":string, "data":variant} {"命令"="", "data"=variant} ("元素"), "命令"="debug", "data"=w521) -> (w524:cluster{"命令":string, "data":variant})
        n321 = Enqueue Element(queue=w527, element=w524) -> ()  [unwired: 2 in, 3 out]
      }
      event "停止": Value Change {
        n322 = event-data() -> ()  [unwired: 1 in, 6 out]
        n323 = Enqueue Element(queue=w531, element=cluster{"命令":string, "data":variant} {"命令"="启动", "data"=variant(cluster{"站号":u16, "控制命令输出":u16[]} {"站号"=1, "控制命令输出"=[2816]})} ("元素")) -> (queue out=w528:refnum<queue>)  [unwired: 2 in, 2 out]
        n324 = Enqueue Element(queue=w528, element=cluster{"命令":string, "data":variant} {"命令"="启动", "data"=variant(cluster{"站号":u16, "控制命令输出":u16[]} {"站号"=2, "控制命令输出"=[2816]})} ("元素")) -> ()  [unwired: 2 in, 3 out]
      }
      event "设置": Value Change {
        n325 = event-data() -> ()  [unwired: 1 in, 6 out]
        n326 = property on="窗格" class="Pane"("Origin"=T10 {"Horizontal"=0, "Vertical"=628} ("原点")) -> ()  [unwired: 2 in, 2 out]
      }
      event "返回": Value Change {
        n327 = event-data() -> ()  [unwired: 1 in, 6 out]
        n328 = property on="窗格" class="Pane"("Origin"=T10 {"Horizontal"=0, "Vertical"=0} ("原点")) -> ()  [unwired: 2 in, 2 out]
      }
      event "公式.X^2", "公式.X", "公式.b", "量程切换阈值.阈值", "量程切换阈值.标液浓度", "备用系数.量程上限", "备用系数.量程下限", "备用系数.检出限", "备用系数.精度", "总氮稀释倍数": Mouse Down {
        n329 = event-data() -> ("CtlRef"=w537:refnum<vi>)  [unwired: 1 in, 5 out]
        n330 = property class="DigNum (严格)"(reference=w537) -> (reference out=w535:refnum<vi>, "Value"=w536:dbl)  [unwired: 1 in, 1 out]
        n331 = call "数字键盘.vi"("OldNumber"=w536) -> ("NewNumber"=w534:dbl)
        n332 = property class="DigNum (严格)"(reference=w535, "Val(Sgnl)"=w534) -> ()  [unwired: 1 in, 2 out]
      }
      event "读公式": Value Change {
        n333 = event-data() -> ()  [unwired: 1 in, 6 out]
        n334 = property class="Enum (严格)"(reference=w545) -> ("Value"=w544:enum16{"总磷", "总氮"})  [unwired: 1 in, 2 out]
        n335 = property class="Enum (严格)"(reference=w546) -> ("Value"=w543:enum16{"水样测量", "空白核查", "跨度核查", "标样核查", "加标回收"})  [unwired: 1 in, 2 out]
        n336 = property class="Enum (严格)"(reference=w547) -> ("Value"=w542:enum16{"低量程", "高量程"})  [unwired: 1 in, 2 out]
        n337 = call "总磷总氮公式读取.vi"("量程"=w542, "测量模式"=w543, "测量参数"=w544) -> ("error out"=w539:errorcluster, "公式"=w540:cluster{"X^2":dbl, "X":dbl, "b":dbl})  [unwired: 7 in]
        n338 = property class="Clust (严格)"(reference=w541, "Value"=w540) -> ()  [unwired: 1 in, 2 out]
        n339 = case shown="错误" w539 {
          tunnel: ["读取成功" ("消息") "读取失败" ("消息")] -> w538
          frame No Error {
          }
          frame Error {
          }
        }
        n340 = One Button Dialog(message=w538) -> ()  [unwired: 1 in, 1 out]
      }
      event "写公式": Value Change {
        n341 = event-data() -> ()  [unwired: 1 in, 6 out]
        n342 = call "总磷总氮公式写入.vi"("公式"="公式", "量程"="量程下拉列表", "测量模式"="测量模式下拉列表", "测量参数"="参数下拉列表") -> ("error out"=w552:errorcluster)  [unwired: 7 in]
        n343 = case shown="无错误" w552 {
          tunnel: ["写入成功" ("消息") "写入失败" ("消息")] -> w553
          frame No Error {
          }
          frame Error {
          }
        }
        n344 = One Button Dialog(message=w553) -> ()  [unwired: 1 in, 1 out]
      }
      event "量程切换阈值读取": Value Change {
        n345 = event-data() -> ()  [unwired: 1 in, 6 out]
        n346 = property class="Enum (严格)"(reference=w565) -> ("Value"=w564:enum16{"总磷", "总氮"})  [unwired: 1 in, 2 out]
        n347 = property class="Enum (严格)"(reference=w566) -> ("Value"=w563:enum16{"水样测量", "空白核查", "跨度核查", "标样核查", "加标回收"})  [unwired: 1 in, 2 out]
        n348 = property class="Enum (严格)"(reference=w567) -> ("Value"=w562:enum16{"低量程", "高量程"})  [unwired: 1 in, 2 out]
        n349 = call "总磷总氮量程读取.vi"("量程"=w562, "测量模式"=w563, "测量参数"=w564) -> ("error out"=w558:errorcluster, "量程切换阈值"=w560:cluster{"阈值":dbl, "标液浓度":dbl})  [unwired: 7 in]
        n350 = property class="Clust (严格)"(reference=w561, "Value"=w560) -> ()  [unwired: 1 in, 2 out]
        n351 = case shown="错误" w558 {
          tunnel: ["读取成功" ("消息") "读取失败" ("消息")] -> w559
          frame No Error {
          }
          frame Error {
          }
        }
        n352 = One Button Dialog(message=w559) -> ()  [unwired: 1 in, 1 out]
      }
      event "量程切换阈值写入": Value Change {
        n353 = event-data() -> ()  [unwired: 1 in, 6 out]
        n354 = property class="Enum (严格)"(reference=w578) -> ("Value"=w575:enum16{"总磷", "总氮"})  [unwired: 1 in, 2 out]
        n355 = property class="Enum (严格)"(reference=w577) -> ("Value"=w574:enum16{"水样测量", "空白核查", "跨度核查", "标样核查", "加标回收"})  [unwired: 1 in, 2 out]
        n356 = property class="Enum (严格)"(reference=w576) -> ("Value"=w573:enum16{"低量程", "高量程"})  [unwired: 1 in, 2 out]
        n357 = call "总磷总氮量程写入.vi"("量程切换阈值"="量程切换阈值", "量程"=w573, "测量模式"=w574, "测量参数"=w575) -> ("error out"=w570:errorcluster)  [unwired: 7 in]
        n358 = case shown="无错误" w570 {
          tunnel: ["写入成功" ("消息") "写入失败" ("消息")] -> w571
          frame No Error {
          }
          frame Error {
          }
        }
        n359 = One Button Dialog(message=w571) -> ()  [unwired: 1 in, 1 out]
      }
      event "备用系数读取": Value Change {
        n360 = event-data() -> ()  [unwired: 1 in, 6 out]
        n361 = property class="Enum (严格)"(reference=w586) -> ("Value"=w585:enum16{"总磷", "总氮"})  [unwired: 1 in, 2 out]
        n362 = call "总磷总氮备用系数读取.vi"("测量参数"=w585) -> ("error out"=w581:errorcluster, "备用系数"=w583:T2)  [unwired: 9 in]
        n363 = property class="Clust (严格)"(reference=w584, "Value"=w583) -> ()  [unwired: 1 in, 2 out]
        n364 = case shown="错误" w581 {
          tunnel: ["读取成功" ("消息") "读取失败" ("消息")] -> w582
          frame No Error {
          }
          frame Error {
          }
        }
        n365 = One Button Dialog(message=w582) -> ()  [unwired: 1 in, 1 out]
      }
      event "备用系数写入": Value Change {
        n366 = event-data() -> ()  [unwired: 1 in, 6 out]
        n367 = property class="Enum (严格)"(reference=w593) -> ("Value"=w592:enum16{"总磷", "总氮"})  [unwired: 1 in, 2 out]
        n368 = call "总磷总氮备用系数写入.vi"("备用系数"="备用系数", "测量参数"=w592) -> ("error out"=w589:errorcluster)  [unwired: 9 in]
        n369 = case shown="无错误" w589 {
          tunnel: ["写入成功" ("消息") "写入失败" ("消息")] -> w590
          frame No Error {
          }
          frame Error {
          }
        }
        n370 = One Button Dialog(message=w590) -> ()  [unwired: 1 in, 1 out]
      }
    }
  }
